vi "Pump 2 Alone.vi"() -> ()   [LabVIEW 2013]
uses:
  <vilib>/rvi/interface/common/niFpgaWaitOnOcc.vi
  <vilib>/FPGAPlugInAG/sbRIO-9642/niLvFpga_Open_sbRIO-9642.vi
  <vilib>/rvi/interface/common/dynamic/niFpgaDynamicAddResources.vi
  <vilib>/Utility/error.llb/Error Cluster From Error Code.vi
  <vilib>/rvi/errors/niLvFpgaAdjustHostInterfaceError.vi
  <vilib>/rvi/interface/nirviOpenFPGA/nirviOpenFPGA.xnode
  FPGA Bitfiles/TCO2TestingProje_FPGATarget_MicrofluidicsFPG_1krVi7I6L8M.lvbitx
  FPGA Code/Microfluidics FPGA Control.vi
  <vilib>/rvi/interface/nirviReadWriteControl/nirviReadWriteControl.xnode
  <vilib>/rvi/interface/Simulation/niFpgaSimulationCallBeginRW.vi
  NiFpgaLv.dll
panel:
  in  "P2 Steps":i32=500
  in  "P2 Speed":dbl=20.0
  in  "P2 Direction":bool=TRUE
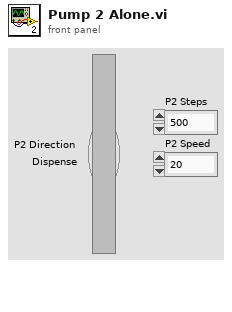
[diagram p1: front panel]
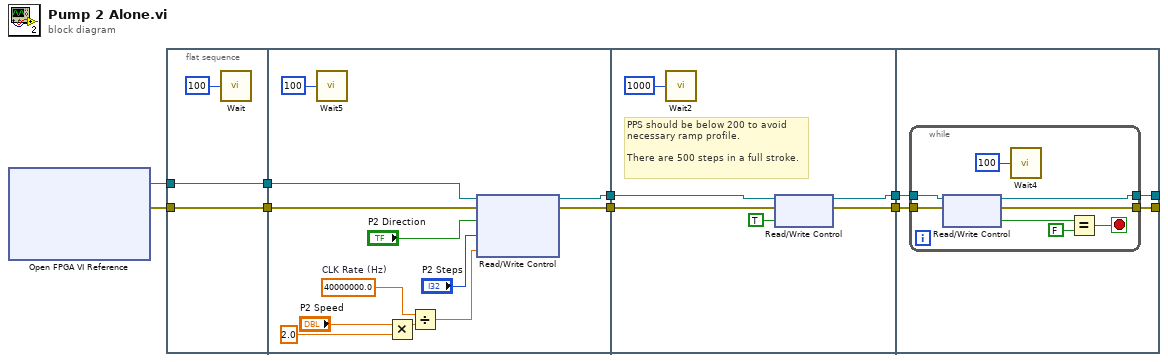
[diagram p0: block diagram]
diagram:
  n1 = xnode "Open FPGA VI Reference"() -> ("FPGA VI Reference Out"=w8:refnum<k20>, "error out"=w7:errorcluster)  [unwired: 2 in]
  n2 = flat-sequence {
    tunnel: w7 -> [w10]
    tunnel: w8 -> [w11]
    tunnel: [w11] -> w4
    tunnel: [w10] -> w2
    tunnel: w4 -> [w19]
    tunnel: [w22] -> w3
    tunnel: w2 -> [w20]
    tunnel: [w23] -> w1
    tunnel: [w26] -> w5
    tunnel: [w25] -> w6
    tunnel: w3 -> [w28]
    tunnel: w1 -> [w27]
    tunnel: w6 -> [w33]
    tunnel: w5 -> [w32]
    tunnel: [w31] -> _
    tunnel: [w30] -> _
    frame #0 {
      n3 = call "Wait"("Count(mSec)"=u32 100) -> ()  [unwired: 1 out]
    }
    frame #1 {
      w17 = 40000000.0  # CLK Rate (Hz)
      n4 = call "Wait5"("Count(mSec)"=u32 100) -> ()  [unwired: 1 out]
      n5 = Multiply(x="P2 Speed", y=2.0) -> (x*y=w13:dbl)
      n6 = Divide(x=w17, y=w13) -> (x/y=w14:dbl)
      n7 = xnode "Read/Write Control"("FPGA VI Reference In"=w19, "error in"=w20, "P2 Direction"="P2 Direction", "P2 Steps"="P2 Steps", "P2 Period"=w14) -> ("FPGA VI Reference Out"=w22:refnum<k20>, "error out"=w23:errorcluster)
    }
    frame #2 {
      # "PPS should be below 200 to avoid \nnecessary ramp profile.\n\nThere are 500 steps in a full stroke."
      n8 = call "Wait2"("Count(mSec)"=u32 1000) -> ()  [unwired: 1 out]
      n9 = xnode "Read/Write Control"("FPGA VI Reference In"=w28, "error in"=w27, "Start P2"=TRUE ("Pump 2 PWR")) -> ("FPGA VI Reference Out"=w25:refnum<k20>, "error out"=w26:errorcluster)
    }
    frame #3 {
      n10 = while {
        tunnel: w33 -> [w41]
        tunnel: w32 -> [w40]
        tunnel: [w39] -> w31
        tunnel: [w38] -> w30
        stop <- w34 stop-if-true
        n11 = xnode "Read/Write Control"("FPGA VI Reference In"=w41, "error in"=w40) -> ("FPGA VI Reference Out"=w39:refnum<k20>, "error out"=w38:errorcluster, "Start P2"=w36:bool)
        n12 = call "Wait4"("Count(mSec)"=u32 100) -> ()  [unwired: 1 out]
        n13 = Equal?(x=w36, y=FALSE) -> (x = y?=w34:bool)
      }
    }
  }
